vi "srecS3Parse.vi"(11 "SrecS3":string="S0130000537461746963566972656F2E73726563A4\nS30D00000000000000B0500008B832\nS30D00000008000000B0483308B8FF\nS30D00000010000000B0044108B82D\nS30D00000020000000B0A00308B8BF\nS31500000050000000B0584EA031000000B0904840307B\nS31500000060000000B0E8562030000000B08402F4B969\nS3150000007000000080000000B0141EF4B90000A33098\nS31500000080000000B8000000B0544EA030000000B0E0\nS31500000090574E803006006030002085140318441641\nS315000000A00C0052BC08000FB600000080000000B033\nS315000000B000006030F0FF03BCE4FF21300000E1F9EE\nS315000000C00018FC99000000800000E1E908000FB666\nS315000000D01C002130000000B0544EA030000000B0DB\nS315000000...") -> (3 "DataRecord":cluster{"Address":u32, "Data":u32}[](array[cluster]) {"Address" format="%.0x"; "Data" format="%.0x"})   [LabVIEW 2015]
panel:
  out "NumElements":i32
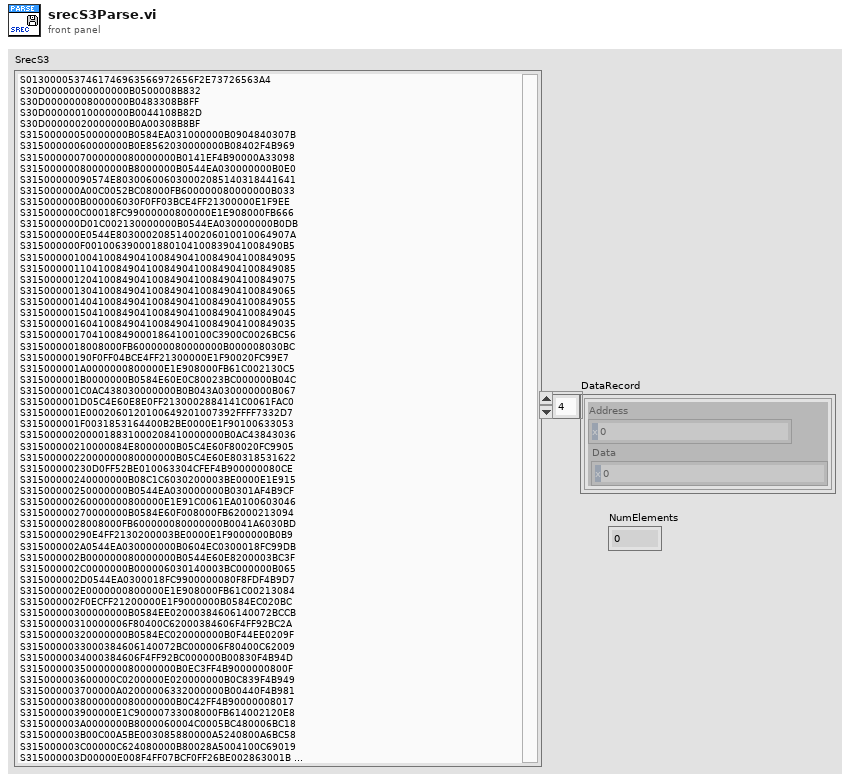
[diagram p1: front panel]
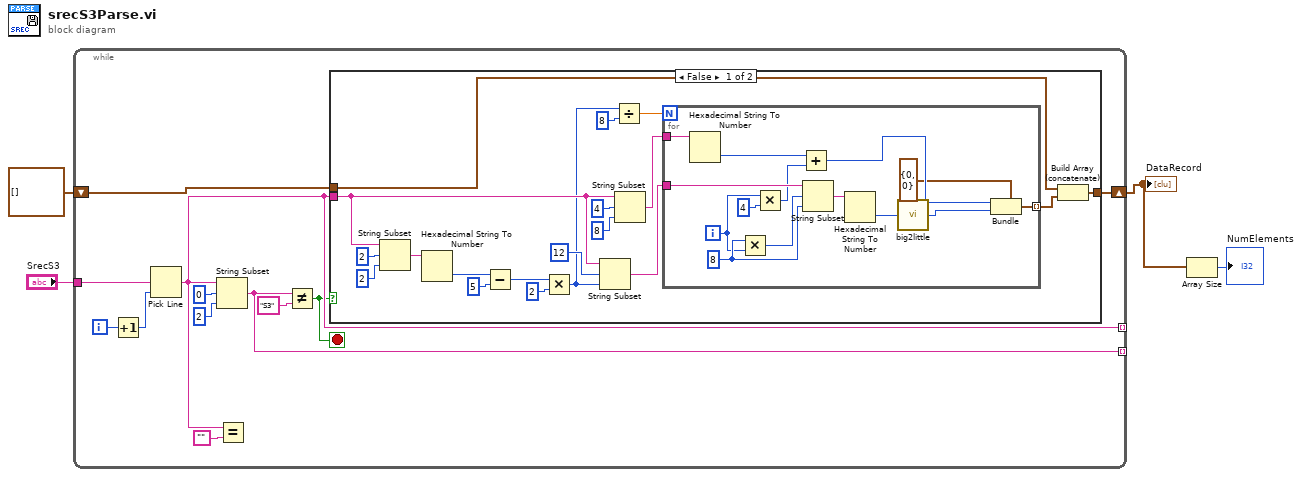
[diagram p0: block diagram]
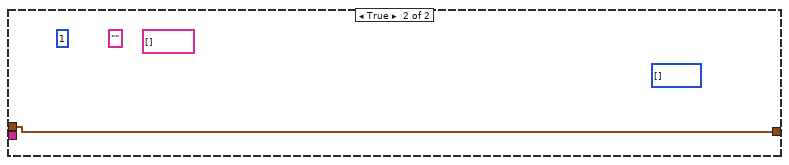
[diagram p2: hidden frame]
diagram:
  n1 = while {
    tunnel: [w9] -> _ mode=indexing
    tunnel: [w11] -> _ mode=indexing
    tunnel: "SrecS3" -> [w7]
    shift-right: [w6] -> w3
    shift-left: cluster{"Address":u32, "Data":u32}[] [] -> [w5]
    i -> [w15]
    stop <- w8 stop-if-true
    n2 = Increment(x=w15) -> (x+1=w14:i32)
    n3 = Pick Line(multi-line string=w7, line index=w14) -> (output string=w9:string)  [unwired: 1 in]
    n4 = String Subset(string=w9, offset (0)=0, length (rest)=2 ("length (rest)")) -> (substring=w11:string)
    n5 = Equal?(x=w9, y="") -> ()  [unwired: 1 out]
    n6 = Not Equal?(x=w11, y="S3") -> (x != y?=w8:bool)
    n7 = case shown="False" w8 {
      tunnel: w9 -> [w26 _]
      tunnel: [w19 w50] -> w6
      tunnel: w5 -> [w18 w50]
      frame False {
        n8 = String Subset(string=w26, offset (0)=2, length (rest)=2 ("length (rest)")) -> (substring=w31:string)
        n9 = Hexadecimal String To Number(string=w31) -> (number=w30:u32)  [unwired: 2 in, 1 out]
        n10 = Subtract(x=w30, y=u32 5) -> (x-y=w27:u32)
        n11 = Multiply(x=w27, y=u32 2) -> (x*y=w24:u32)
        n12 = String Subset(string=w26, offset (0)=12, length (rest)=w24) -> (substring=w21:string)
        n13 = Divide(x=w24, y=u32 8) -> (x/y=w22:dbl)
        n14 = String Subset(string=w26, offset (0)=4, length (rest)=8 ("length (rest)")) -> (substring=w20:string)
        n15 = for {
          N: w22 -> [_]
          tunnel: w21 -> [w49]
          tunnel: w20 -> [w46]
          tunnel: [w37] -> w17 mode=indexing
          i -> [w45]
          w47 = 8 ("length (rest)")
          n16 = Hexadecimal String To Number(string=w46) -> (number=w42:u32)  [unwired: 2 in, 1 out]
          n17 = Multiply(x=w47, y=w45) -> (x*y=w48:i32)
          n18 = Multiply(x=w45, y=4) -> (x*y=w44:i32)
          n19 = Add(x=w42, y=w44) -> (x+y=w39:u32)
          n20 = String Subset(string=w49, offset (0)=w48, length (rest)=w47) -> (substring=w41:string)
          n21 = Hexadecimal String To Number(string=w41) -> (number=w40:u32)  [unwired: 2 in, 1 out]
          n22 = call "big2little.vi"("BigEndian"=w40) -> ("SmallEndian"=w38:u32)
          n23 = Bundle(cluster=cluster{"Address":u32, "Data":u32} {"Address"=0, "Data"=0}, "Address"=w39, "Data"=w38) -> (w37:cluster{"Address":u32, "Data":u32})
        }
        n24 = Build Array (concatenate)(w18, w17) -> (w19:cluster{"Address":u32, "Data":u32}[])
      }
      frame True {
        (unwired) i32[] []
        (unwired) string[] []
        (unwired) u32 1
        (unwired) "" ("output string")
      }
    }
  }
  "DataRecord" <- w3
  n25 = Array Size(array=w3) -> (size(s)=→"NumElements":i32)
